vi "Write.vi"(8 "error in (no error)":errorcluster, 9 "Variant":variant, 10 "String":string, 11 "AK RS232 in":refnum<class "AK RS-xxx.lvclass">) -> (0 "error out":errorcluster, 3 "AK RS232 out":refnum<class "AK RS-xxx.lvclass">)   [LabVIEW 2023, in "Protocols.lvlib" / "AK RS-xxx.lvclass"]
uses:
  AK RS-xxx.lvclass
  RS-xxx/RS-xxx.lvclass
  Protocols.lvlib
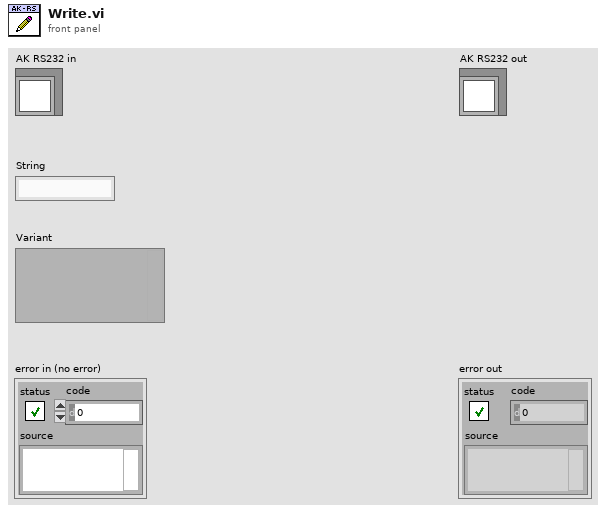
[diagram p1: front panel]
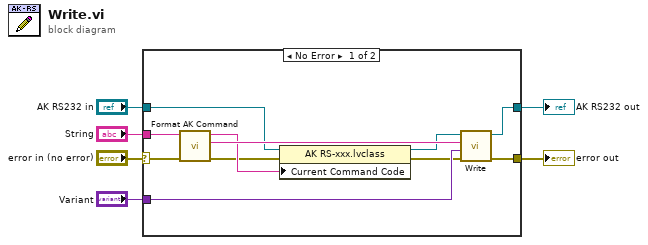
[diagram p0: block diagram]
diagram:
  n1 = case shown="No Error" "error in (no error)" {
    selector: "error in (no error)" -> [w7 w19]
    tunnel: [w17 w19] -> w6
    tunnel: [w16 w18] -> w5
    tunnel: "Variant" -> [w15 _]
    tunnel: "String" -> [w13 _]
    tunnel: "AK RS232 in" -> [w12 w18]
    frame No Error {
      n2 = call "Format AK Command.vi"("error in (no error)"=w7, "String in"=w13) -> ("error out"=w8:errorcluster, "Command"=w14:string, "Command Code"=w9:string)  [unwired: 7 in]
      n3 = property class="AK RS-xxx.lvclass"(reference=w12, error in=w8, "Current Command Code"=w9) -> (reference out=w11:refnum<class "AK RS-xxx.lvclass">, error out=w10:errorcluster)
      n4 = call-parent "Write.vi"("error in (no error)"=w10, "Variant"=w15, "String"=w14, "RS232 in"=w11) -> ("error out"=w17:errorcluster, "RS232 out"=w16:refnum<class "AK RS-xxx.lvclass">)  [unwired: 6 in]
    }
    frame Error {
    }
  }
  "error out" <- w6
  "AK RS232 out" <- w5
